vi "Error.vi"(0 "User Message (A fault has been detected.)":string="A fault has been detected.", 7 "Clear Error (T)":bool=TRUE, 11 "error in (no error)":errorcluster) -> (8 "Error":bool=TRUE, 15 "error out":errorcluster)   [LabVIEW 2021]
panel:
  out "Error Detail":string caption="Technical Information"
  out "Error Summary":string
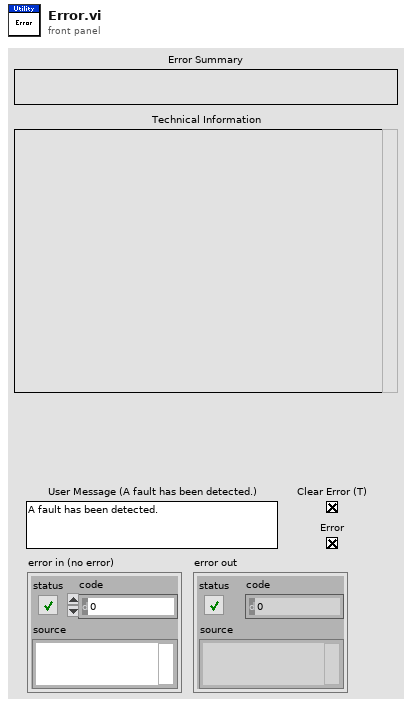
[diagram p1: front panel]
types:
  T1 = enum32{"Invalid", "Standard", "Closed", "Hidden", "Minimized", "Maximized"}
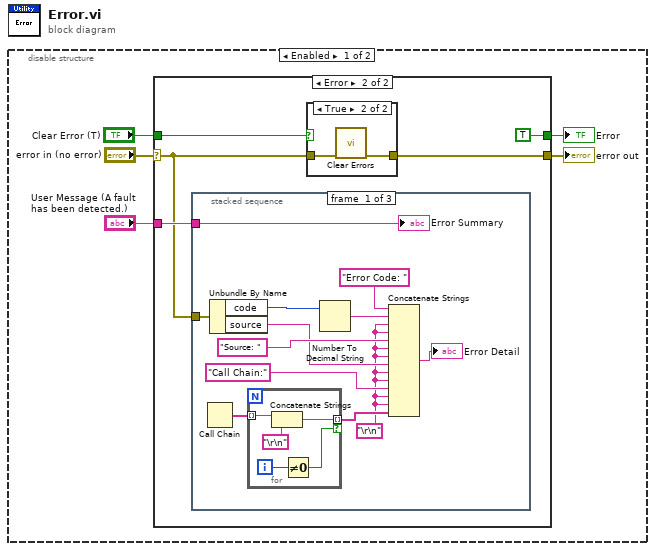
[diagram p0: block diagram]
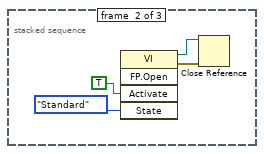
[diagram p4: hidden frame]
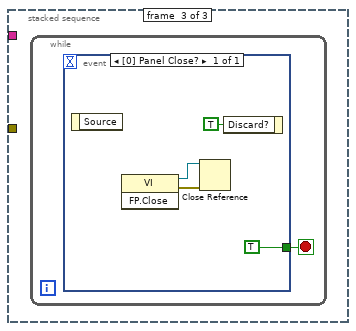
[diagram p5: hidden frame]
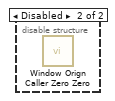
[diagram p6: hidden frame]
diagram:
  n1 = disable-structure shown="Enabled" {
    frame Enabled {
      n2 = case shown="Error" "error in (no error)" {
        selector: "error in (no error)" -> [w6 w9]
        tunnel: [w6 w10] -> w4
        tunnel: "User Message (A fault has been detected.)" -> [_ w11]
        tunnel: "Clear Error (T)" -> [_ w8]
        tunnel: [_ TRUE ("No Error")] -> w1
        frame No Error {
        }
        frame Error {
          n3 = stacked-sequence {
            tunnel: w9 -> [w26 _ _]
            tunnel: w11 -> [w25 _ _]
            frame #0 {
              w15 = "\r\n"
              n4 = Call Chain() -> (call chain=w18:string[])
              n5 = Unbundle By Name(w26) -> ("code"=w24:i32, "source"=w19:string)
              n6 = for {
                tunnel: w18 -> [w31] mode=indexing
                tunnel: [w29] -> w17 mode=indexing if=w27
                i -> [w28]
                n7 = Concatenate Strings(w31, "\r\n") -> (w29:string)
                n8 = Not Equal To 0?(x=w28) -> (x != 0?=w27:bool)
              }
              n9 = Number To Decimal String(number=w24) -> (decimal integer string=w23:string)  [unwired: 1 in]
              n10 = Concatenate Strings("Error Code: ", w23, w15, w15, "Source: " ("string"), w15, w15, w19, w15, w15, "Call Chain:" ("string"), w15, w15, w17) -> (→"Error Detail":string)
              "Error Summary" <- w25
            }
            frame #1 {
              n11 = invoke class="VI" method="FP.Open"("Activate"=TRUE ("Activate?"), "State"=T1."Standard") -> (reference out=w35:refnum<vi>, error out=w34:errorcluster)  [unwired: 3 in, 3 out]
              n12 = Close Reference(reference=w35, error in (no error)=w34) -> ()  [unwired: 1 out]
            }
            frame #2 {
              n13 = while {
                stop <- w36 stop-if-true
                n14 = event shown="[0] Panel Close?" {
                  selector: _ -> [_]
                  dyn-events: _ -> [_]
                  timeout: _ -> [_]
                  tunnel: [TRUE] -> w36
                  event Panel Close? {
                    n15 = event-data() -> ()  [unwired: 1 in, 1 out]
                    n16 = invoke class="VI" method="FP.Close"() -> (reference out=w37:refnum<vi>, error out=w38:errorcluster)  [unwired: 3 in, 1 out]
                    n17 = Close Reference(reference=w37, error in (no error)=w38) -> ()  [unwired: 1 out]
                    n18 = event-data("Discard?"=TRUE) -> ()  [unwired: 1 in, 1 out]
                  }
                }
              }
            }
          }
          n19 = case shown="True" w8 {
            tunnel: [w12 w14] -> w10
            tunnel: w9 -> [w12 w13]
            frame False {
            }
            frame True {
              n20 = call <vilib>:"Clear Errors.vi"("error in (no error)"=w13) -> ("error out"=w14:errorcluster)  [unwired: 5 in, 1 out]
            }
          }
        }
      }
      "error out" <- w4
      "Error" <- w1
    }
    frame Disabled {
      n21 = call "Window Orign Caller Zero Zero.vi"() -> ()  [unwired: 15 in, 1 out]
    }
  }
